vi "SubVI_ControlIntakePosition_Intake.vi"(9 "(IntakeDown)":bool, 10 "(IntakeUp)":bool) -> (2 "IntakePosition":dbl)   [LabVIEW 2017]
uses:
  <vilib>/Rock Robotics/Network Tables/NT Read Number.vi
  <vilib>/Rock Robotics/Network Tables/NT Write Number.vi
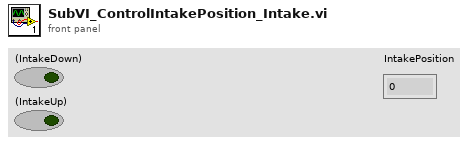
[diagram p1: front panel]
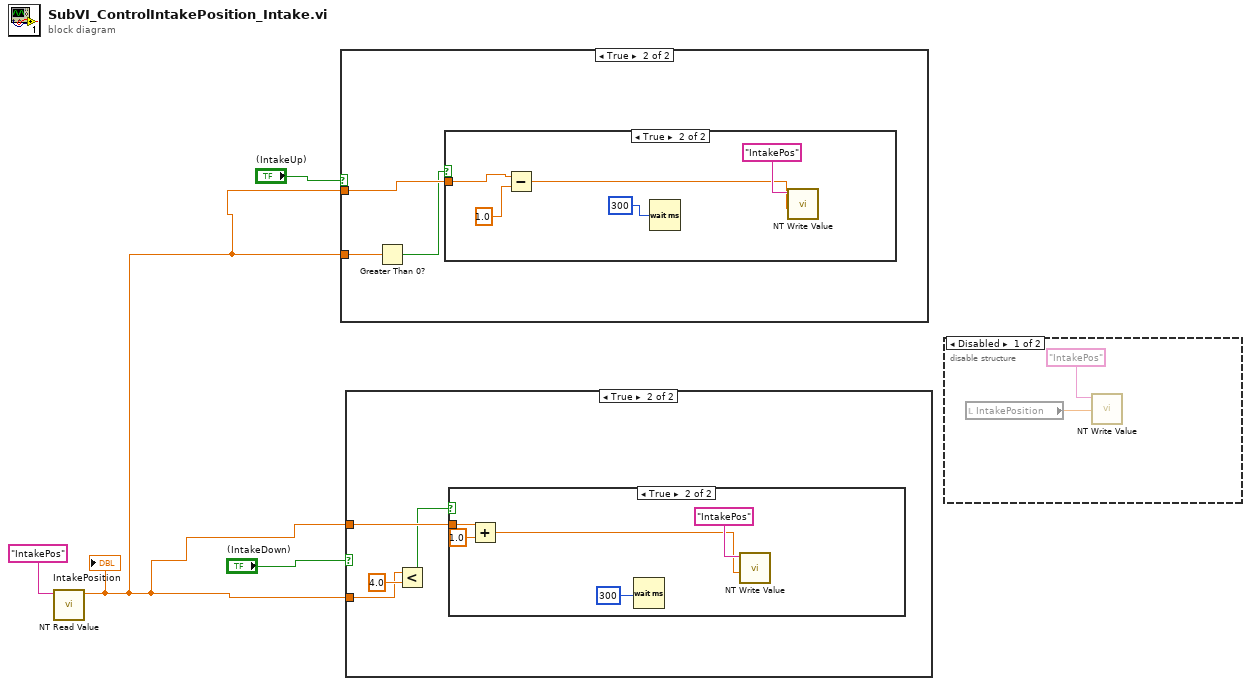
[diagram p0: block diagram]
diagram:
  n1 = call-poly <vilib>:"NT Read Value.vi"("Name"="IntakePos") -> ("Numeric"=w3:dbl)  [unwired: 9 in, 1 out]
  "IntakePosition" <- w3
  n2 = case shown="True" "(IntakeUp)" {
    tunnel: w3 -> [_ w7]
    tunnel: w3 -> [_ w6]
    frame False {
    }
    frame True {
      n3 = Greater Than 0?(x=w6) -> (x > 0?=w5:bool)
      n4 = case shown="True" w5 {
        tunnel: w7 -> [_ w12]
        frame False {
        }
        frame True {
          n5 = Subtract(x=w12, y=1.0) -> (x-y=w8:dbl)
          n6 = Wait (ms)(milliseconds to wait=u32 300) -> ()  [unwired: 1 out]
          n7 = call-poly <vilib>:"NT Write Value.vi"("Numeric"=w8, "Name"="IntakePos") -> ()  [unwired: 9 in, 1 out]
        }
      }
    }
  }
  n8 = case shown="True" "(IntakeDown)" {
    tunnel: w3 -> [_ w14]
    tunnel: w3 -> [_ w15]
    frame False {
    }
    frame True {
      n9 = Less?(x=w15, y=4.0) -> (x < y?=w13:bool)
      n10 = case shown="True" w13 {
        tunnel: w14 -> [_ w18]
        frame False {
        }
        frame True {
          n11 = Add(x=w18, y=1.0) -> (x+y=w17:dbl)
          n12 = Wait (ms)(milliseconds to wait=u32 300) -> ()  [unwired: 1 out]
          n13 = call-poly <vilib>:"NT Write Value.vi"("Numeric"=w17, "Name"="IntakePos") -> ()  [unwired: 9 in, 1 out]
        }
      }
    }
  }
  n14 = disable-structure shown="Disabled" {
    frame Disabled {
      n15 = local read "IntakePosition"() -> (w22:dbl)
      n16 = call-poly <vilib>:"NT Write Value.vi"("Numeric"=w22, "Name"="IntakePos") -> ()  [unwired: 9 in, 1 out]
    }
    frame Enabled {
    }
  }
